vi "Send Calibrate Potentiometers.vi"(7 "Priority":T2=enum."Normal" caption="Message Priority (Normal)", 8 "error in (no error)":errorcluster, 9 "rate":dbl=1000.0 format="%0.2f", 10 "DAQ  Channels In":T1={"Force Transducer: Left"="Dev1/ai6", "Force Transducer: Right "="Dev1/ai8", "EMG: Left"="", "EMG: Right"="", "Potentiometer: Left"="", "Potentiometer: Right"=""}, 11 "Message Enqueuer in":refnum<class "Message Enqueuer.lvclass">) -> (0 "error out":errorcluster, 3 "Message Enqueuer out":refnum<class "Message Enqueuer.lvclass">)   [LabVIEW 2020, in "NI Force Task.lvlib" / "Calibrate Potentiometers Msg.lvclass"]
doc: "Sends the <b>Calibrate Potentiometers Msg.lvclass</b> message.\n\nThis message will call <b>Calibrate Potentiometers.vi</b> on the <b>NI Force Task.lvlib:NI Force Task.lvclass</b> actor.\n\n<b>Calibrate Potentiometers.vi Description</b>"
uses:
  Calibrate Potentiometers Msg.lvclass
  <vilib>/ActorFramework/Message Enqueuer/Message Enqueuer.lvclass
  <vilib>/ActorFramework/Message Enqueuer/Message Priority.ctl
  C:/Program Files/National Instruments/LabVIEW 2020/vi.lib/ActorFramework/Message/Message.lvclass
  Calibrate Potentiometers Msg.lvclass/Calibrate Potentiometers Msg.ctl
  <vilib>/ActorFramework/Message Enqueuer/Message Enqueuer.lvclass/Message Enqueuer.ctl
  <vilib>/ActorFramework/Message Priority Queue/Priority Enqueue.vi
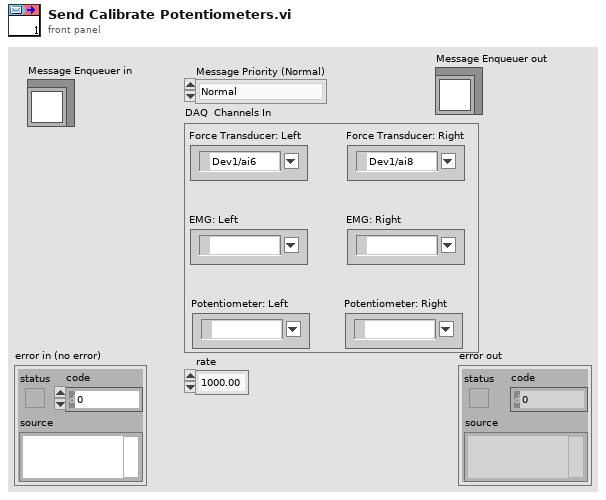
[diagram p1: front panel]
types:
  T1 = cluster{"Force Transducer: Left":tag, "Force Transducer: Right ":tag, "EMG: Left":tag, "EMG: Right":tag, "Potentiometer: Left":tag, "Potentiometer: Right":tag}
  T2 = typedef "Actor Framework.lvlib/Message Enqueuer.lvclass/Message Priority.ctl" = enum16{"Low", "Normal", "High"}
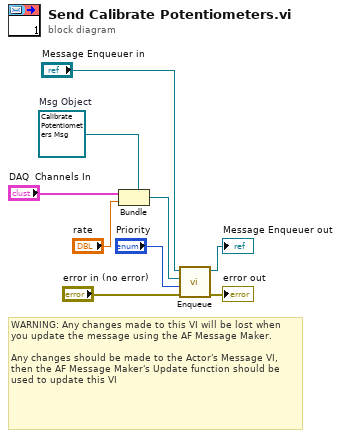
[diagram p0: block diagram]
diagram:
  w7 = refnum<class "Calibrate Potentiometers Msg.lvclass"> refnum  # Msg Object
  # "WARNING: Any changes made to this VI will be lost when you update the message using the AF Message Maker.\n\nAny changes should be made to the Actor's Message VI, then the AF Message Maker's Update function should be used to update this VI"
  n1 = Bundle(cluster=w7, "DAQ  Channels In", "rate") -> (w2:refnum<class "Calibrate Potentiometers Msg.lvclass">)
  n2 = call <vilib>:"Enqueue.vi"("error in (no error)"="error in (no error)", "Message Priority (Normal)"="Priority", "Message"=w2, "Message Enqueuer in"="Message Enqueuer in") -> ("error out"=→"error out":errorcluster, "Message Enqueuer out"=→"Message Enqueuer out":refnum<class "Message Enqueuer.lvclass">)  [unwired: 6 in]
